vi "Test Invalid Multiple Channels Registration - Mismatched Arrays.vi"() -> ()   [LabVIEW 2024]
uses:
  Mock Sift Proxy Server/Mock Sift Proxy Server.lvclass
  Sift API/Sift Client.lvclass
  Sift API/Types/Data Type.ctl
  Sift Client.lvlib
panel:
  out "Server Error":errorcluster
  out "Success":bool
  out "Error 2":errorcluster
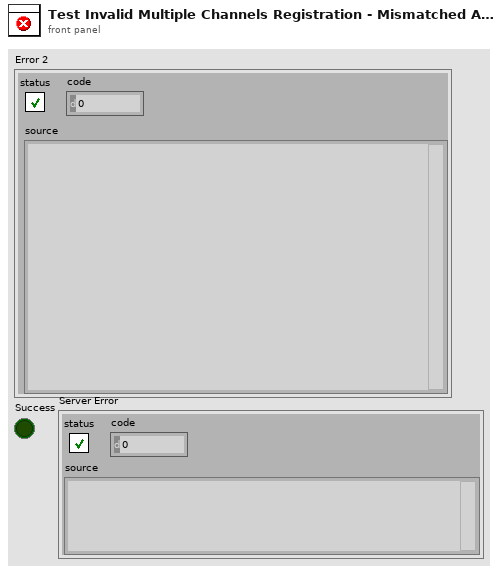
[diagram p1: front panel]
types:
  T1 = typedef "Sift Client.lvlib/Data Type.ctl" = enum8{"double", "float", "uint64", "int64", "uint32", "int32", "bool", "bit field", "enum"}
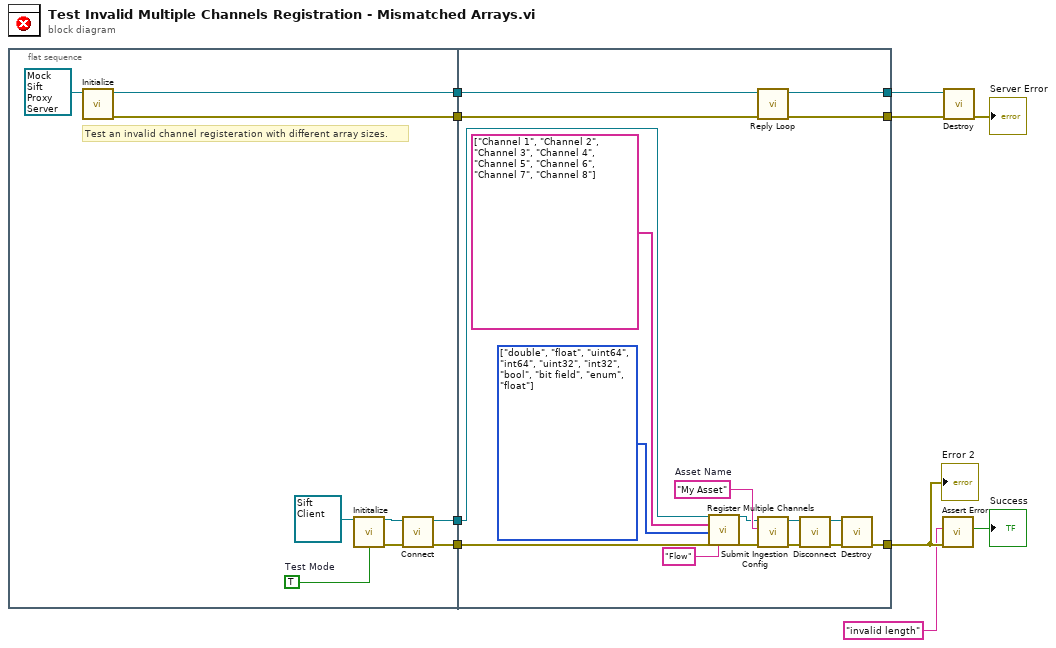
[diagram p0: block diagram]
diagram:
  n1 = flat-sequence {
    tunnel: [w18] -> w10
    tunnel: [w13] -> w9
    tunnel: [w12] -> w8
    tunnel: [w11] -> w7
    tunnel: [w28] -> w5
    tunnel: w10 -> [w29]
    tunnel: [w34] -> w4
    tunnel: w9 -> [w27]
    tunnel: w8 -> [w26]
    tunnel: w7 -> [w23]
    tunnel: [w22] -> w3
    frame #0 {
      w16 = TRUE  # Test Mode
      # "Test an invalid channel registeration with different array sizes."
      n2 = call-dynamic "Initialize.vi"("Mock Sift Proxy Server in"=refnum<class "Mock Sift Proxy Server.lvclass"> refnum ("Mock Sift Proxy Server.lvclass")) -> ("error out"=w11:errorcluster, "Mock Sift Proxy Server out"=w18:refnum<class "Mock Sift Proxy Server.lvclass">)  [unwired: 9 in]
      n3 = call-dynamic "Inititalize.vi"("Sift Client in"=refnum<class "Sift Client.lvclass"> refnum ("Sift Client.lvlib:Sift Client.lvclass"), "Test Mode"=w16) -> ("Sift Client out"=w14:refnum<class "Sift Client.lvclass">, "error out"=w15:errorcluster)  [unwired: 12 in]
      n4 = call-dynamic "Connect.vi"("error in (no error)"=w15, "Sift Client in"=w14) -> ("error out"=w13:errorcluster, "Sift Client out"=w12:refnum<class "Sift Client.lvclass">)  [unwired: 7 in, 1 out]
    }
    frame #1 {
      w20 = T1[] [enum."double", enum."float", enum."uint64", enum."int64", enum."uint32", enum."int32", enum."bool", enum."bit field", enum."enum", enum."float"] items=["double", "float", "uint64", "int64", "uint32", "int32", "bool", "bit field", "enum"]
      w33 = "My Asset"  # Asset Name
      n5 = call "Register Multiple Channels.vi"("Sift Client in"=w26, "Names"=string[] ["Channel 1", "Channel 2", "Channel 3", "Channel 4", "Channel 5", "Channel 6", "Channel 7", "Channel 8"], "Data Types"=w20, "error in (no error)"=w27, "Flow Name"="Flow") -> ("Sift Client out"=w31:refnum<class "Sift Client.lvclass">, "error out"=w35:errorcluster)  [unwired: 21 in]
      n6 = call-dynamic "Reply Loop.vi"("error in (no error)"=w23, "Mock Sift Proxy Server in"=w29) -> ("error out"=w22:errorcluster, "Mock Sift Proxy Server out"=w28:refnum<class "Mock Sift Proxy Server.lvclass">)  [unwired: 8 in]
      n7 = call-dynamic "Submit Ingestion Config.vi"("error in (no error)"=w35, "Asset Name"=w33, "Sift Client in"=w31) -> ("error out"=w36:errorcluster, "Sift Client out"=w30:refnum<class "Sift Client.lvclass">)  [unwired: 7 in]
      n8 = call-dynamic "Disconnect.vi"("error in (no error)"=w36, "Sift Client in"=w30) -> ("error out"=w24:errorcluster, "Sift Client out"=w25:refnum<class "Sift Client.lvclass">)  [unwired: 8 in]
      n9 = call-dynamic "Destroy.vi"("error in (no error)"=w24, "Sift Client in"=w25) -> ("error out"=w34:errorcluster)  [unwired: 8 in, 1 out]
    }
  }
  n10 = call "Assert Error.vi"("Error"=w4, "Error String"="invalid length") -> ("Success"=→"Success":bool)  [unwired: 9 in]
  n11 = call-dynamic "Destroy.vi"("error in (no error)"=w3, "Mock Sift Proxy Server in"=w5) -> ("error out"=→"Server Error":errorcluster)  [unwired: 8 in, 1 out]
  "Error 2" <- w4
